vi "Apply Tab.vi"(0 "MulticolumnListbox in":refnum<vi>, 5 "f":i32, 7 "Columns":T1[](array[typedef])) -> ()   [LabVIEW 2015, in "KTable.xctl"]
uses:
  KTable.xctl
  ColumnType.ctl
  ColumnSpec.ctl
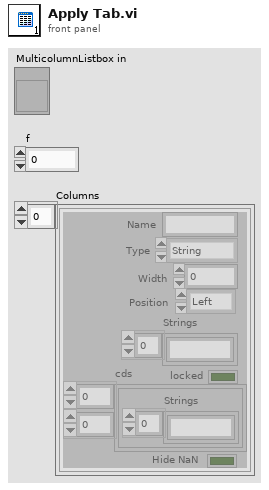
[diagram p1: front panel]
types:
  T1 = typedef "KTable.xctl/ColumnSpec.ctl" = cluster{"Name":string, "Type":T2, "Width":i32, "Strings":string[], "Position":enum16{"Left", "Center", "Right"}, "locked":bool, "cds":cluster{"Strings":string[]}[][], "Hide NaN":bool}
  T2 = typedef "KTable.xctl/ColumnType.ctl" = enum16{"String", "Enum", "Int", "Double", "Boolean", "Ring", "Formula", "Color"}
  T3 = typedef "LVRowAndColumnTypeDef.ctl" = cluster{"Row":i32, "Column":i32}
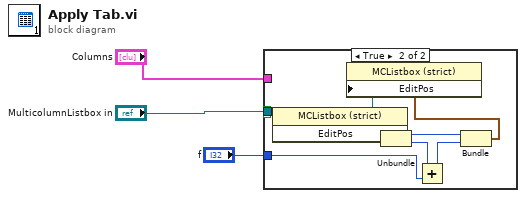
[diagram p0: block diagram]
diagram:
  n1 = case shown="True" {
    selector: _ -> [_ _]
    tunnel: "MulticolumnListbox in" -> [_ w11]
    tunnel: "f" -> [_ w4]
    tunnel: "Columns" -> [_ _]
    frame False {
    }
    frame True {
      n2 = property class="MCListbox (strict)"(reference=w11) -> (reference out=w6:refnum<vi>, "EditPos"=w7:T3)  [unwired: 1 in, 1 out]
      n3 = Unbundle(w7) -> ("Row"=w8:i32, "Column"=w9:i32)
      n4 = Add(x=w9, y=w4) -> (x+y=w10:i32)
      n5 = Bundle("Row"=w8, w10) -> (w5:cluster{"Row":i32, i32})  [unwired: 1 in]
      n6 = property class="MCListbox (strict)"(reference=w6, "EditPos"=w5) -> ()  [unwired: 1 in, 2 out]
    }
  }
